vi "Extract Element JSON.vi"(11 "Ctl Refnum in":refnum<vi>) -> (0 "JSON":string, 1 "Type":string, 2 "Is GUI Element":bool, 3 "Ctl Refnum":refnum<vi>)   [LabVIEW 2020, in "VolatusGUIControls.lvlib"]
uses:
  74616f74-1830-4ff5-a2b6-8e366ce61fd3.vi
  <vilib>/JDP Science/JSONtext/Next JSON Value.vi
  <vilib>/JDP Science/JSONtext/String Subset.vi
  <vilib>/JDP Science/JSONtext/Parsing/Advance past next JSON Value (inlined COPY).vi
  <vilib>/JDP Science/JSONtext/Parsing/Advance past whitespace.vi
  <vilib>/JDP Science/JSONtext/Parsing/Advance past String.vi
  <vilib>/JDP Science/JSONtext/Parsing/Advance past Number.vi
  <vilib>/JDP Science/JSONtext/Parsing/Advance past Line Ending.vi
  <vilib>/JDP Science/JSONtext/Parsing/Parse Full Path or Item Name.vi
  <vilib>/JDP Science/JSONtext/Parsing/Advance past Array.vi
  <vilib>/JDP Science/JSONtext/Parsing/Advance past Object.vi
  <vilib>/JDP Science/JSONtext/support/Error Cluster From Code.vi
  <vilib>/JDP Science/JSONtext/Offset/Find Item Locations by Path.vi
  <vilib>/JDP Science/JSONtext/JSON text to Variant.vi
  <vilib>/JDP Science/JSONtext/LVClass Serializer/JSONtext LVClass Serializer.lvclass
  VolatusGUIControls/VolatusGUIControls.lvlib
  <vilib>/JDP Science/JSONtext/JSONtext.lvlib
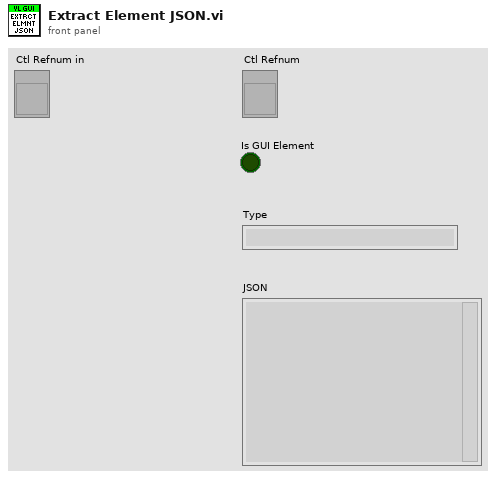
[diagram p1: front panel]
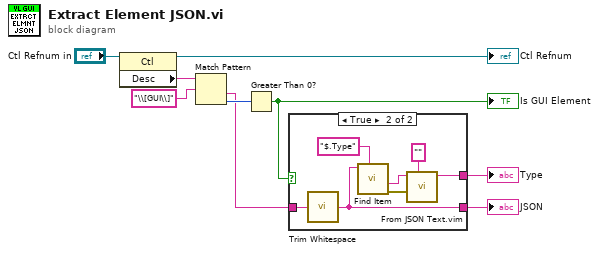
[diagram p0: block diagram]
diagram:
  n1 = property class="Ctl"(reference="Ctl Refnum in") -> (reference out=→"Ctl Refnum":refnum<vi>, "Desc"=w9:string)  [unwired: 1 in, 1 out]
  n2 = Match Pattern(string=w9, regular expression="\\[GUI\\]") -> (after substring=w3:string, offset past match=w7:i32)  [unwired: 1 in, 2 out]
  n3 = Greater Than 0?(x=w7) -> (x > 0?=w4:bool)
  "Is GUI Element" <- w4
  n4 = case shown="True" w4 {
    tunnel: w3 -> [_ w16]
    tunnel: [_ w11] -> w2
    tunnel: [_ w10] -> w1
    frame False {
    }
    frame True {
      n5 = call <vilib>:"Trim Whitespace.vi"("string"=w16) -> ("trimmed string"=w10:string)  [unwired: 1 in]
      n6 = call <vilib>:"Find Item.vi"("$Path or Item Name"="$.Type", "JSON"=w10) -> ("error out"=w14:errorcluster, "<JSON>"=w13:string)  [unwired: 6 in, 2 out]
      n7 = call "From JSON Text.vim"("Data Type and Default Value"="", "error in (no error)"=w14, "JSON"=w13) -> ("Data out"=w11:string)  [unwired: 7 in, 1 out]
    }
  }
  "Type" <- w2
  "JSON" <- w1
